vi "CreateWriteHDF5File.vi"(5 "Enum":enum16{"CAMERA", "PMT"}(ring), 6 "string seq in":string, 7 "pmt data in":u64[][](array[numeric]), 8 "error in (no error)":errorcluster, 9 "path":path, 10 "attributes":T1, 11 "Data in camera":i32[][][][](array[numeric])) -> (0 "error out":errorcluster)   [LabVIEW 2019]
uses:
  <vilib>/Utility/miscctls.llb/LVRectTypeDef.ctl
  <vilib>/UPVI/lvhdf5/group.llb/H5G_obj_t.ctl
  <vilib>/UPVI/lvhdf5/dataset.llb/LVH5D Operation.ctl
  <vilib>/UPVI/lvhdf5/group.llb/OpenCreateGroup (String).vi
  <vilib>/Utility/VariantDataType/GetClusterInfo.vi
  <vilib>/Utility/VariantDataType/GetTypeInfo.vi
  <vilib>/UPVI/lvhdf5/attribute.llb/Write Multiple Attributes.vi
  <vilib>/UPVI/lvhdf5/utility.llb/Select HDF5 Dialog.vi
  <vilib>/UPVI/lvhdf5/utility.llb/Select HDF5 Dialog (Object Only).vi
  <vilib>/UPVI/lvhdf5/dataset.llb/Simple H5Dwrite (Variant).vi
  <vilib>/Utility/file.llb/Read From Spreadsheet File (DBL).vi
  <vilib>/UPVI/lvhdf5/attribute.llb/Simple H5Awrite (Variant).vi
  <vilib>/UPVI/lvhdf5/attribute.llb/LVH5A Operation.ctl
  <vilib>/UPVI/lvhdf5/attribute.llb/LVH5 Write Attributes.xnode
  <vilib>/UPVI/lvhdf5/library.llb/HDF5 Ref.ctl
  <vilib>/UPVI/lvhdf5/attribute.llb/Cluster to Attribute Array.xnode
  <vilib>/UPVI/lvhdf5/dataset.llb/Simple H5Dwrite.xnode
  <vilib>/UPVI/lvhdf5/Attribute.llb/Simple H5Awrite.xnode
  <vilib>/UPVI/lvhdf5/identifier.llb/Not an HDF5 Refnum Constant.vi
  <vilib>/Utility/error.llb/Error Cluster From Error Code.vi
  <vilib>/UPVI/lvhdf5/dataset.llb/OpenCreateReplace Dataset by Element Type.vi
  <vilib>/UPVI/lvhdf5/dataspace.llb/H5Sselect_hyperslab.vi
  <vilib>/UPVI/lvhdf5/dataset.llb/H5Dwrite (Variant).vi
  <vilib>/UPVI/lvhdf5/dataset.llb/H5Dget_space.vi
  <vilib>/UPVI/lvhdf5/attribute.llb/private/LVH5AwriteWDTAttrs.vi
  <vilib>/UPVI/lvhdf5/dataspace.llb/H5Sclose.vi
  <vilib>/UPVI/lvhdf5/dataset.llb/H5Dclose.vi
  <vilib>/UPVI/lvhdf5/file.llb/OpenCreateReplace HDF5 File.vi
  <vilib>/UPVI/lvhdf5/file.llb/LVH5F Operation.ctl
  <vilib>/UPVI/lvhdf5/utility.llb/Select HDF5 Dialog (File and Object).vi
  <vilib>/Utility/VariantDataType/VariantType.lvlib
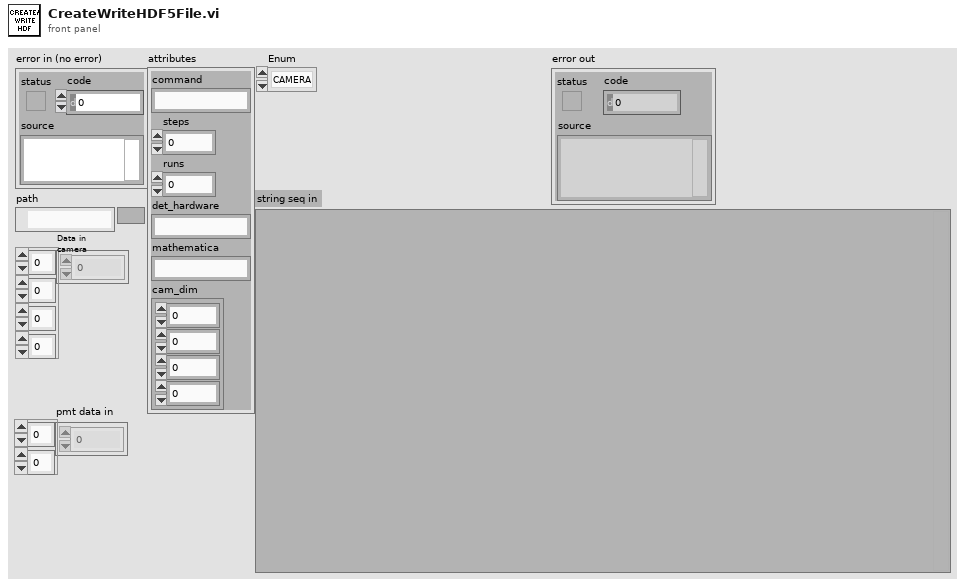
[diagram p1: front panel]
types:
  T1 = cluster{"command":string, "steps":dbl, "runs":dbl, "det_hardware":string, "mathematica":string, "cam_dim":cluster{i32, i32, i32, i32}}
  T2 = typedef "HDF5 Ref.ctl" = refnum<k1>
  T3 = typedef "LVRectTypeDef.ctl" = cluster{"Left":i16, "Top":i16, "Right":i16, "Bottom":i16}
  T4 = cluster{"Behavior":enum32{"Invalid", "Default", "Floating", "Floating/Auto-Hide", "Modal"}, "Position":T3, "Center":bool, "Title":string}
  T5 = typedef "LVH5F Operation.ctl" = enum16{"open", "open or create", "create or replace", "create or replace (with confirmation)", "create", "open (read only)"}
  T6 = typedef "LVH5D Operation.ctl" = enum16{"open", "replace", "create", "open or create", "create or replace", "create or replace with confirmation"}
  T7 = typedef "H5G_obj_t.ctl" = i32
  T8 = cluster{"Object Types (any)":T7[], "Object Pattern":string}
  T9 = cluster{"t1":i32, "t2":i32, "errm1":string, "errm2":string}
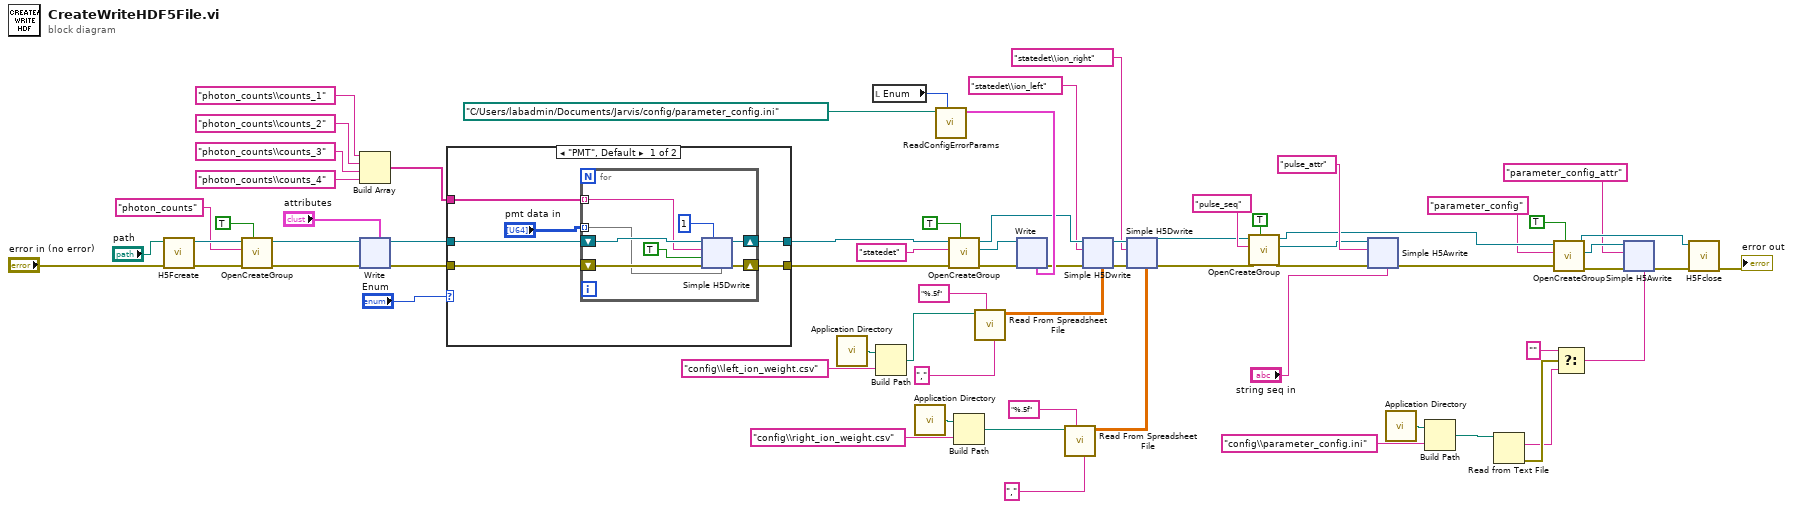
[diagram p0: block diagram]
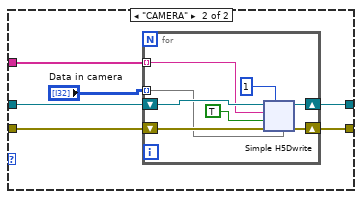
[diagram p2: hidden frame]
diagram:
  n1 = call <vilib>:"H5Fcreate.vi"("error in (no error)"="error in (no error)", "path"="path") -> ("error out"=w68:errorcluster, "HDF5 Ref"=w69:T2)  [unwired: 6 in]
  n2 = call-poly <vilib>:"OpenCreateGroup.vi"("Create if not found (F)"=TRUE, "error in (no error)"=w68, "Group"="photon_counts", "HDF5 Ref"=w69) -> ("error out"=w52:errorcluster, "HDF5 Ref out"=w53:T2)  [unwired: 5 in, 1 out]
  n3 = Build Array("photon_counts\\counts_1" ("Dataset Path"), "photon_counts\\counts_2" ("Dataset Path"), "photon_counts\\counts_3" ("Dataset Path"), "photon_counts\\counts_4" ("Dataset Path")) -> (w29:string[])
  n4 = xnode "Write"("HDF5 Ref"=w53, "error in (no error)"=w52, "Value(s)"="attributes") -> ("HDF5 Ref out"=w51:T2, "error out"=w50:errorcluster)  [unwired: 2 in]
  n5 = case shown="\"PMT\", Default" "Enum" {
    tunnel: w51 -> [w75 w291]
    tunnel: w50 -> [w74 w290]
    tunnel: w29 -> [w73 w289]
    tunnel: [w72 w288] -> w28
    tunnel: [w71 w287] -> w27
    frame "PMT", Default {
      n6 = for {
        shift-right: [w79] -> w71
        shift-left: w74 -> [w81]
        shift-right: [w78] -> w72
        shift-left: w75 -> [w82]
        tunnel: w73 -> [w76] mode=indexing
        tunnel: "pmt data in" -> [w77] mode=indexing
        n7 = xnode "Simple H5Dwrite"("Compression Level (0-disabled)"=1, "Dataset Path"=w76, "Unlimited  dataset (F)"=TRUE, "error in (no error)"=w81, "HDF5 Path or Ref"=w82, "Data"=w77) -> ("HDF5 Ref out"=w78:T2, "error out"=w79:errorcluster)  [unwired: 2 in, 1 out]
      }
    }
    frame "CAMERA" {
      n8 = for {
        shift-right: [w295] -> w287
        shift-left: w290 -> [w297]
        shift-right: [w294] -> w288
        shift-left: w291 -> [w298]
        tunnel: w289 -> [w292] mode=indexing
        tunnel: "Data in camera" -> [w293] mode=indexing
        n9 = xnode "Simple H5Dwrite"("Compression Level (0-disabled)"=1, "Dataset Path"=w292, "Unlimited  dataset (F)"=TRUE, "error in (no error)"=w297, "HDF5 Path or Ref"=w298, "Data"=w293) -> ("HDF5 Ref out"=w294:T2, "error out"=w295:errorcluster)  [unwired: 2 in, 1 out]
      }
    }
  }
  n10 = call <vilib>:"Application Directory.vi"() -> ("Application Directory"=w47:path)
  n11 = local read "Enum"() -> (w25:enum16{"CAMERA", "PMT"})
  n12 = Build Path(base path=w47, name or relative path="config\\left_ion_weight.csv") -> (appended path=w46:path)
  n13 = call <vilib>:"Application Directory.vi"() -> ("Application Directory"=w42:path)
  n14 = call "ReadConfigErrorParams.vi"("hardware"=w25, "configuration file path"=path "C:/Users/labadmin/Documents/Jarvis/config/parameter_config.ini") -> ("err_params"=w60:T9)  [unwired: 9 in]
  n15 = call-poly <vilib>:"OpenCreateGroup.vi"("Create if not found (F)"=TRUE, "error in (no error)"=w27, "Group"="statedet", "HDF5 Ref"=w28) -> ("error out"=w61:errorcluster, "HDF5 Group Ref"=w62:T2, "HDF5 Ref out"=w59:T2)  [unwired: 5 in]
  n16 = Build Path(base path=w42, name or relative path="config\\right_ion_weight.csv") -> (appended path=w41:path)
  n17 = call-poly <vilib>:"Read From Spreadsheet File.vi"("delimiter (\\t)"="," ("delimiter (\\t)"), "format (%.3f)"="%.5f", "file path (dialog if empty)"=w46) -> ("all rows"=w49:dbl[][])  [unwired: 4 in, 4 out]
  n18 = xnode "Write"("HDF5 Ref"=w62, "error in (no error)"=w61, "Value(s)"=w60) -> ("error out"=w58:errorcluster)  [unwired: 2 in, 1 out]
  n19 = call-poly <vilib>:"Read From Spreadsheet File.vi"("delimiter (\\t)"="," ("delimiter (\\t)"), "format (%.3f)"="%.5f", "file path (dialog if empty)"=w41) -> ("all rows"=w38:dbl[][])  [unwired: 4 in, 4 out]
  n20 = xnode "Simple H5Dwrite"("Dataset Path"="statedet\\ion_left", "error in (no error)"=w58, "HDF5 Path or Ref"=w59, "Data"=w49) -> ("HDF5 Ref out"=w56:T2, "error out"=w55:errorcluster)  [unwired: 4 in, 1 out]
  n21 = xnode "Simple H5Dwrite"("Dataset Path"="statedet\\ion_right", "error in (no error)"=w55, "HDF5 Path or Ref"=w56, "Data"=w38) -> ("HDF5 Ref out"=w22:T2, "error out"=w21:errorcluster)  [unwired: 4 in, 1 out]
  n22 = call-poly <vilib>:"OpenCreateGroup.vi"("Create if not found (F)"=TRUE, "error in (no error)"=w21, "Group"="pulse_seq", "HDF5 Ref"=w22) -> ("error out"=w19:errorcluster, "HDF5 Group Ref"=w18:T2, "HDF5 Ref out"=w6:T2)  [unwired: 5 in]
  n23 = xnode "Simple H5Awrite"("HDF5 Ref"=w18, "Name"="pulse_attr", "error in (no error)"=w19, "Value"="string seq in") -> ("error out"=w9:errorcluster)  [unwired: 1 in, 1 out]
  n24 = call <vilib>:"Application Directory.vi"() -> ("Application Directory"=w16:path)
  n25 = Build Path(base path=w16, name or relative path="config\\parameter_config.ini") -> (appended path=w14:path)
  n26 = Read from Text File(file (use dialog)=w14) -> (text=w11:string, error out=w12:errorcluster)  [unwired: 3 in, 2 out]
  n27 = call-poly <vilib>:"OpenCreateGroup.vi"("Create if not found (F)"=TRUE, "error in (no error)"=w9, "Group"="parameter_config", "HDF5 Ref"=w6) -> ("error out"=w8:errorcluster, "HDF5 Group Ref"=w5:T2, "HDF5 Ref out"=w4:T2)  [unwired: 5 in]
  n28 = Select(t="", s=w12, f=w11) -> (s? t:f=w13:string)
  n29 = xnode "Simple H5Awrite"("HDF5 Ref"=w5, "Name"="parameter_config_attr", "error in (no error)"=w8, "Value"=w13) -> ("error out"=w7:errorcluster)  [unwired: 1 in, 1 out]
  n30 = call <vilib>:"H5Fclose.vi"("error in (no error)"=w7, "HDF5 Ref"=w4) -> ("error out"=→"error out":errorcluster)  [unwired: 7 in]
